vi "Ejercicio 1.vi"() -> ()   [LabVIEW 2021]
panel:
  in  "Numeric 3":dbl
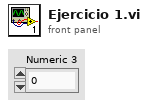
[diagram p1: front panel]
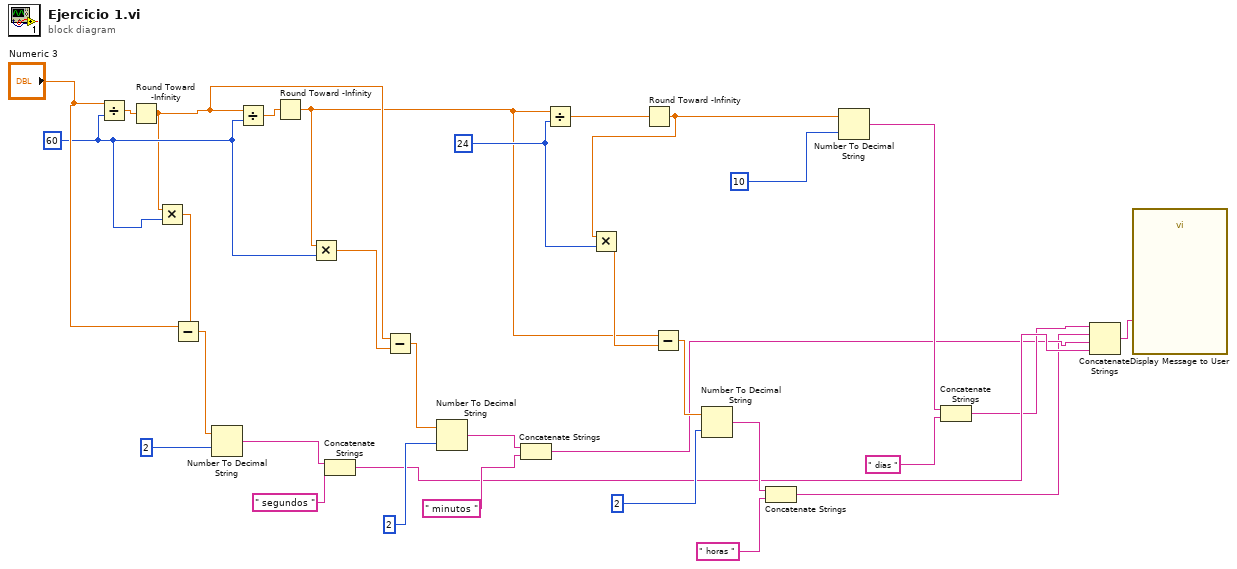
[diagram p0: block diagram]
diagram:
  w31 = 24
  w9 = 60
  n1 = Divide(x="Numeric 3", y=w9) -> (x/y=w10:dbl)
  n2 = Round Toward -Infinity(1:w10) -> (0:w7:dbl)
  n3 = Multiply(x=w7, y=w9) -> (x*y=w8:dbl)
  n4 = Subtract(x="Numeric 3", y=w8) -> (x-y=w14:dbl)
  n5 = Number To Decimal String(number=w14, width (-)=2) -> (decimal integer string=w26:string)
  n6 = Divide(x=w7, y=w9) -> (x/y=w12:dbl)
  n7 = Round Toward -Infinity(1:w12) -> (0:w5:dbl)
  n8 = Multiply(x=w5, y=w9) -> (x*y=w32:dbl)
  n9 = Concatenate Strings(w26, " segundos ") -> (w4:string)
  n10 = Subtract(x=w7, y=w32) -> (x-y=w29:dbl)
  n11 = Number To Decimal String(number=w29, width (-)=2) -> (decimal integer string=w24:string)
  n12 = Concatenate Strings(w24, " minutos ") -> (w2:string)
  n13 = Divide(x=w5, y=w31) -> (x/y=w11:dbl)
  n14 = Round Toward -Infinity(1:w11) -> (0:w6:dbl)
  n15 = Multiply(x=w6, y=w31) -> (x*y=w30:dbl)
  n16 = Subtract(x=w5, y=w30) -> (x-y=w28:dbl)
  n17 = Number To Decimal String(number=w28, width (-)=2) -> (decimal integer string=w23:string)
  n18 = Concatenate Strings(w23, " horas ") -> (w1:string)
  n19 = Number To Decimal String(number=w6, width (-)=10) -> (decimal integer string=w20:string)
  n20 = Concatenate Strings(w20, " días ") -> (w3:string)
  n21 = Concatenate Strings(w3, w1, w2, w4) -> (w15:string)
  n22 = call "Display Message to User"("Message"=w15) -> ()  [unwired: 9 in, 2 out]
